vi "AH2500A Build.vi"() -> ()   [LabVIEW 2019]
uses:
  <vilib>/AppBuilder/AB_API_Simple/Build Specification Version.ctl
  <userlib>/LevyLab/Build Support/PostBuildSupport/PostBuildSupport.lvclass
  <vilib>/MakerHub/Toolbox/LMH-Toolbox.lvlib
  <vilib>/AppBuilder/AB_API_Simple/NI_App_Builder_API.lvlib
  <vilib>/AppBuilder/AB_API_Simple/Set Build Specification Version (path).vi
  <vilib>/AppBuilder/AB_API_Simple/Build (path).vi
panel:
  in  "Package Version (maj.min.fix.build)":string="1.2.0.1"
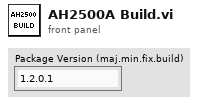
[diagram p1: front panel]
types:
  T1 = typedef "NI_App_Builder_API.lvlib/Build Specification Version.ctl" = cluster{"Major":u16, "Minor":u16, "Fix":u16, "Build":u16}
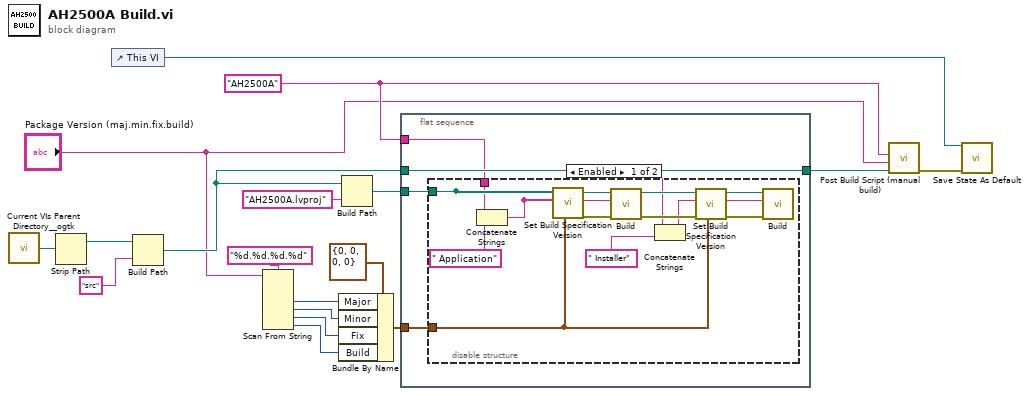
[diagram p0: block diagram]
diagram:
  w4 = "AH2500A" ("Product Name")
  n1 = call <userlib>:"Current VIs Parent Directory__ogtk.vi"() -> ("Parent Directory (+ Relative)"=w18:path)  [unwired: 5 in]
  n2 = Strip Path(path=w18) -> (stripped path=w17:path)  [unwired: 1 out]
  n3 = control-ref of="This VI"() -> (w14:refnum<vi>)
  n4 = Build Path(base path=w17, name or relative path="src") -> (appended path=w3:path)
  n5 = Scan From String(format string="%d.%d.%d.%d", input string="Package Version (maj.min.fix.build)") -> (output 1=w10:i32, output 2=w13:i32, output 3=w9:i32, output 4=w12:i32)  [unwired: 6 in, 3 out]
  n6 = Bundle By Name(cluster=T1 {"Major"=0, "Minor"=0, "Fix"=0, "Build"=0} ("Build Specification Version"), "Major"=w10, "Minor"=w13, "Fix"=w9, "Build"=w12) -> (w7:T1)
  n7 = Build Path(base path=w3, name or relative path="AH2500A.lvproj") -> (appended path=w5:path)
  n8 = flat-sequence {
    tunnel: w7 -> [w22]
    tunnel: w5 -> [w21]
    tunnel: [w20] -> w2
    tunnel: w3 -> [w20]
    tunnel: w4 -> [w19]
    frame #0 {
      n9 = disable-structure shown="Enabled" {
        disable-tunnel: w22 -> [w30 _]
        disable-tunnel: w21 -> [w28 _]
        disable-tunnel: w19 -> [w24 _]
        frame Enabled {
          n10 = Concatenate Strings(w24, " Application" ("Name of build specification")) -> (w26:string)
          n11 = call-poly <vilib>:"Set Build Specification Version.vi"("Build Specification Version"=w30, "Name of build specification"=w26, "Path to project"=w28) -> ("error out"=w32:errorcluster)  [unwired: 8 in]
          n12 = call-poly <vilib>:"Build.vi"("error in (no error)"=w32, "Name of build specification (if empty: build all)"=w26, "Path to project"=w28) -> ("error out"=w31:errorcluster)  [unwired: 7 in, 1 out]
          n13 = Concatenate Strings(w24, " Installer" ("Name of build specification")) -> (w23:string)
          n14 = call-poly <vilib>:"Set Build Specification Version.vi"("Build Specification Version"=w30, "error in (no error)"=w31, "Name of build specification"=w23, "Path to project"=w28) -> ("error out"=w29:errorcluster)  [unwired: 7 in]
          n15 = call-poly <vilib>:"Build.vi"("error in (no error)"=w29, "Name of build specification (if empty: build all)"=w23, "Path to project"=w28) -> ()  [unwired: 7 in, 2 out]
        }
        frame Disabled {
        }
      }
    }
  }
  n16 = call <userlib>:"Post Build Script (manual build).vi"("Package Source Folder"=w2, "Package Version"="Package Version (maj.min.fix.build)", "Product Name"=w4) -> ("error out"=w15:errorcluster)  [unwired: 8 in]
  n17 = call <vilib>:"Save State As Default.vi"("Error In"=w15, "Target VI"=w14) -> ()  [unwired: 8 in, 2 out]
